vi "usrp tx - Copy.vi"() -> ()   [LabVIEW 2014]
uses:
  <instrlib>/niUSRP/niUSRP Write Tx Data (CDB WDT).vi
  <vilib>/Analysis/Matrix/NI_Matrix.lvlib
  <vilib>/Analysis/Matrix/Numeric/Conversions/Matrix To Array - RM.vi
  <vilib>/Analysis/Matrix/Datatypes/RealMatrix.ctl
panel:
  in  "output variable":T1 caption="Real Matrix"
  in  "channel list":string
  in  "Boolean":bool
  out "Waveform Graph":waveform(dbl)(graph)
  in  "active antenna":string
  in  "carrier frequency":dbl=100000.0 format="%#_6p"
  in  "IQ rate":dbl=100000.0 format="%#_6p"
  in  "device names":refnum<k15>
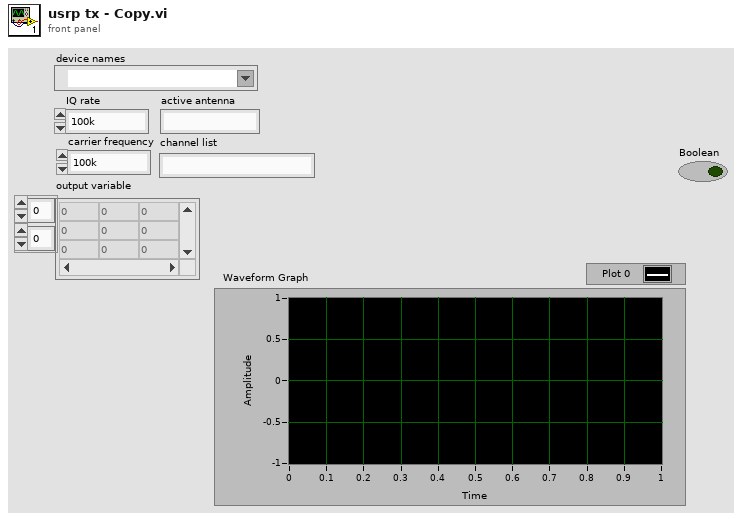
[diagram p1: front panel]
types:
  T1 = typedef "NI_Matrix.lvlib/RealMatrix.ctl" = dbl[][]
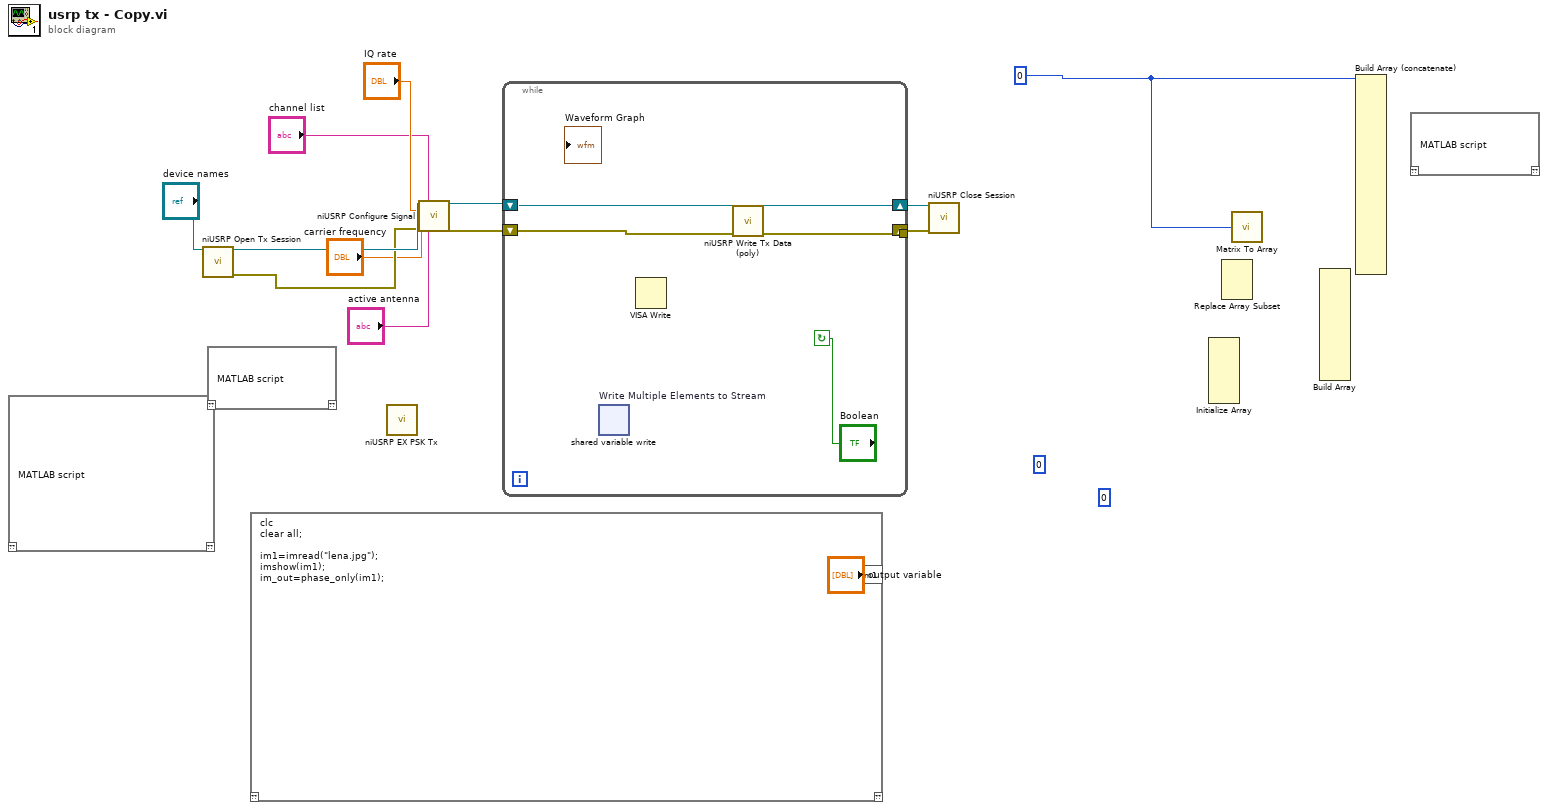
[diagram p0: block diagram]
diagram:
  (unwired) 0
  (unwired) 0
  w2 = 0
  n1 = script code="MATLAB script"() -> ()  [unwired: 1 in, 2 out]
  n2 = call <instrlib>:"niUSRP Open Tx Session.vi"("device names"="device names") -> ("session handle out"=w12:refnum<k15>, "error out"=w11:errorcluster)  [unwired: 13 in]
  n3 = script code="MATLAB script"() -> ()  [unwired: 1 in, 1 out]
  n4 = mathscript code="clc\nclear all;\n\nim1=imread(\"lena.jpg\");\nimshow(im1);\nim_out=phase_only(im1);"() -> ()  [unwired: 2 in, 2 out]
  n5 = call "niUSRP EX PSK Tx.vi"() -> ()  [unwired: 1 in]
  n6 = call <instrlib>:"niUSRP Configure Signal.vi"("session handle"=w12, "channel list"="channel list", "IQ rate"="IQ rate", "carrier frequency"="carrier frequency", "error in (no error)"=w11, "active antenna"="active antenna") -> ("session handle out"=w10:refnum<k15>, "error out"=w9:errorcluster)  [unwired: 5 in, 3 out]
  n7 = while {
    shift-right: [w19] -> w8
    shift-left: w10 -> [w21]
    shift-right: [_] -> w7
    shift-left: w9 -> [w20]
    tunnel: [w16] -> _
    stop <- "Boolean" continue-if-true
    n8 = shared-variable-write "Write Multiple Elements to Stream"() -> ()  [unwired: 4 in, 3 out]
    n9 = VISA Write(write buffer=w15) -> (VISA resource name=w15:refnum<visa-resource-name>)  [unwired: 1 in, 3 out]
    n10 = call-poly <instrlib>:"niUSRP Write Tx Data (poly).vi"("session handle"=w21, "error in (no error)"=w20) -> ("session handle out"=w19:refnum<k15>, "data"=w14:waveform(cdb), "error out"=w16:errorcluster)  [unwired: 11 in]
  }
  n11 = call <instrlib>:"niUSRP Close Session.vi"("session handle"=w8, "error in (no error)"=w7) -> ()  [unwired: 13 in, 1 out]
  n12 = Initialize Array() -> (w1:i32)  [unwired: 6 in, 1 out]
  n13 = Replace Array Subset() -> ()  [unwired: 4 in, 1 out]
  n14 = call-poly <vilib>:"Matrix To Array.vi"("Real 2D Array"=w2) -> ()  [unwired: 1 in]
  n15 = Build Array() -> ()  [unwired: 14 in, 1 out]
  n16 = Build Array (concatenate)(w2) -> ()  [unwired: 24 in, 1 out]
  n17 = script code="MATLAB script"() -> ()  [unwired: 1 in, 1 out]
